vi "ServerPort.vi"(3 "xml content":string) -> (0 "result string":string, 1 "xml content(dup)":string)   [LabVIEW 2013, in "OPCUA XML.lvlib"]
uses:
  OPCUA XML.lvlib
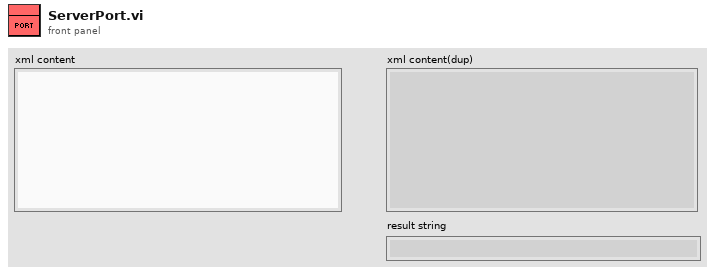
[diagram p1: front panel]
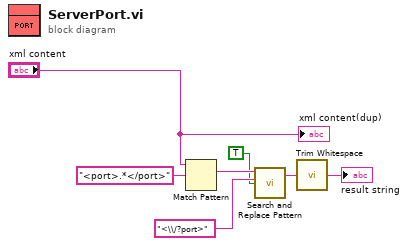
[diagram p0: block diagram]
diagram:
  n1 = Match Pattern(string="xml content", regular expression="<port>.*</port>") -> (match substring=w6:string)  [unwired: 1 in, 3 out]
  n2 = call <vilib>:"Search and Replace Pattern.vi"("string"=w6, "regular expression (\"\")"="<\\/?port>" ("regular expression"), "replace all? (F)"=TRUE) -> ("result string"=w4:string)  [unwired: 2 in, 1 out]
  n3 = call <vilib>:"Trim Whitespace.vi"("string"=w4) -> ("trimmed string"=→"result string":string)  [unwired: 1 in]
  "xml content(dup)" <- "xml content"
